vi "Loop.vi"(7 "Stop Button":bool, 8 "Inputs":T5 {"Color Pane" items=["Blue", "Red", "Green", "Saturation", "Value", "Intensity", "Luminance", "Hue", ""]}, 10 "Reference":T1, 11 "cam5":T6="cam5") -> (0 "Force Cluster":T3, 1 "Diameter Time":dbl, 2 "Force Time":dbl, 3 "Diameter Cluster":T4, 5 "Start Time":timestamp)   [LabVIEW 2020]
uses:
  StateControl.ctl
  <vilib>/vision/driver/NI_Vision_Acquisition_Software.lvlib
  <extravilib>/ChannelInstances/Tag-bool.lvlib
  <vilib>/DAQmx/create/channels.llb/DAQmx Create Channel (AI-Voltage-Basic).vi
  <vilib>/DAQmx/configure/timing.llb/DAQmx Timing (Sample Clock).vi
  <vilib>/DAQmx/write.llb/DAQmx Write (Counter Frequency 1Chan 1Samp).vi
  <vilib>/DAQmx/write.llb/DAQmx Write (Digital Bool 1Line 1Point).vi
  Inputs.ctl
  <vilib>/userDefined/High Color/IMAQdx.ctl
  ButtonReferences.ctl
  BR2.ctl
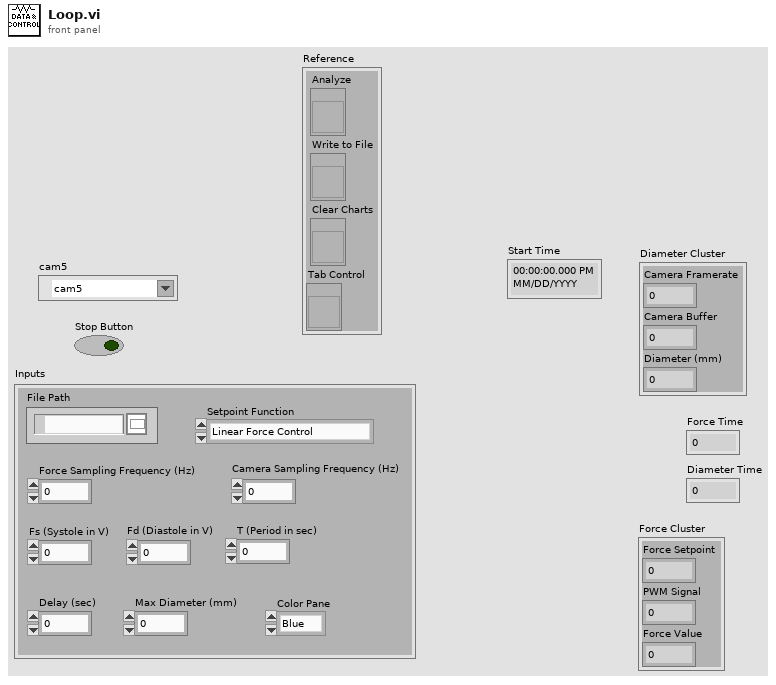
[diagram p1: front panel]
types:
  T1 = typedef "BR2.ctl" = cluster{"Analyze":refnum<vi>, "Write to File":T2, "Clear Charts":refnum<vi>, "Tab Control":refnum<vi>}
  T2 = typedef "ButtonReferences.ctl" = refnum<vi>
  T3 = cluster{"Force Setpoint":dbl, "PWM Signal":dbl, "Force Value":dbl}
  T4 = cluster{"Camera Framerate":dbl, "Camera Buffer":u32, "Diameter (mm)":dbl}
  T5 = typedef "Inputs.ctl" = cluster{"File Path":path, "Force Sampling Frequency (Hz)":dbl, "Camera Sampling Frequency (Hz)":dbl, "Fs (Systole in V)":dbl, "Fd (Diastole in V)":dbl, "T (Period in sec)":dbl, "Delay (sec)":dbl, "Setpoint Function":enum16{"Linear Force Control", "Sinusoidal Force Control", "Blood-Pressure Force Control"}, "Max Diameter (mm)":dbl, "Color Pane":i32}
  T6 = typedef "IMAQdx.ctl" = refnum<k21>
  T7 = typedef "StateControl.ctl" = enum16{"Initialze", "Wait for Event", "Acquire", "Shutdown"}
  T8 = enum8{"Enabled", "Disabled", "Disabled and Grayed Out"}
  T9 = typedef "Image Type" = u32
  T10 = typedef "IMAQ Image.ctl" = refnum<image>
  T11 = typedef "Tag-bool.lvlib/))Channel.ctl" = refnum<queue>
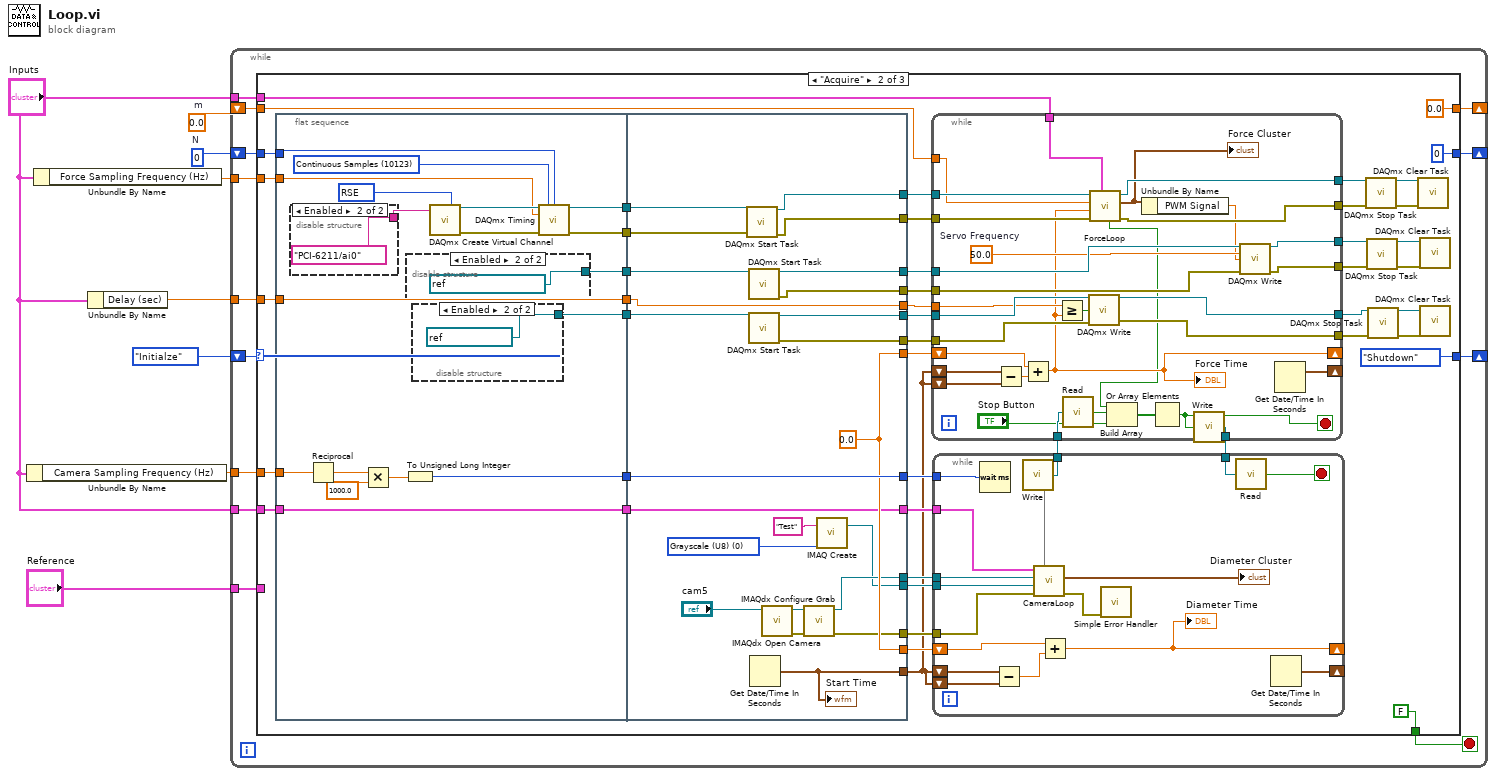
[diagram p0: block diagram]
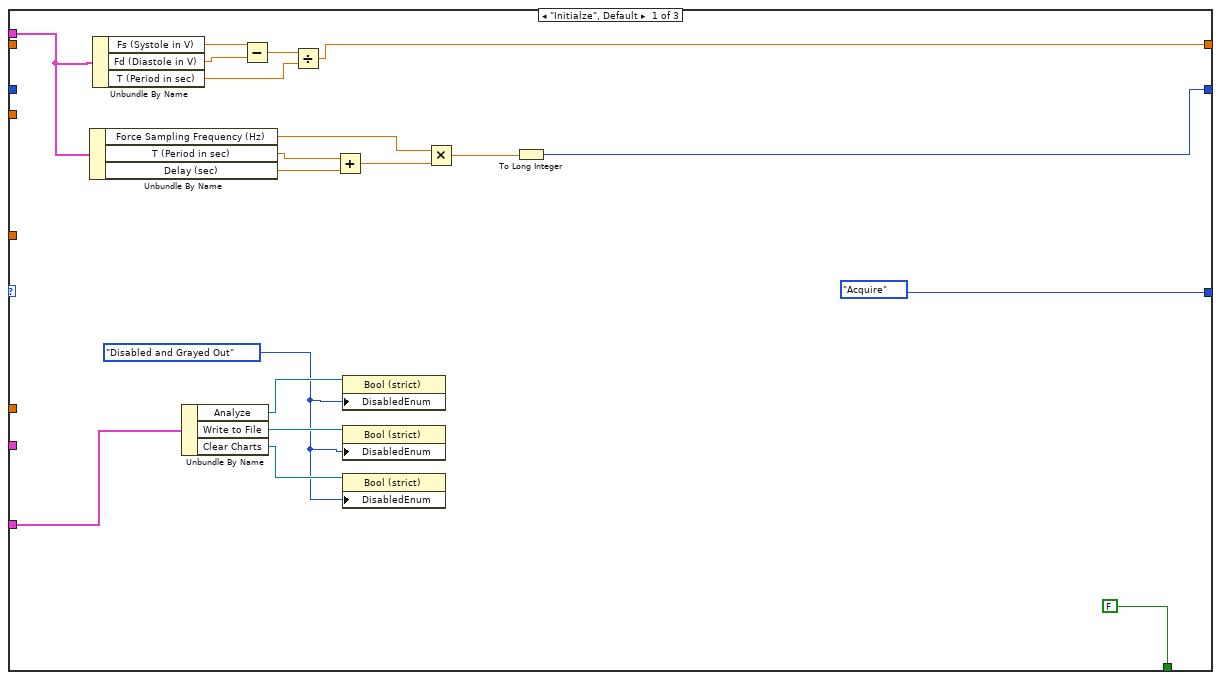
[diagram p2: hidden frame]
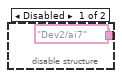
[diagram p3: hidden frame]
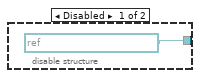
[diagram p4: hidden frame]
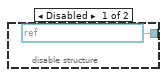
[diagram p5: hidden frame]
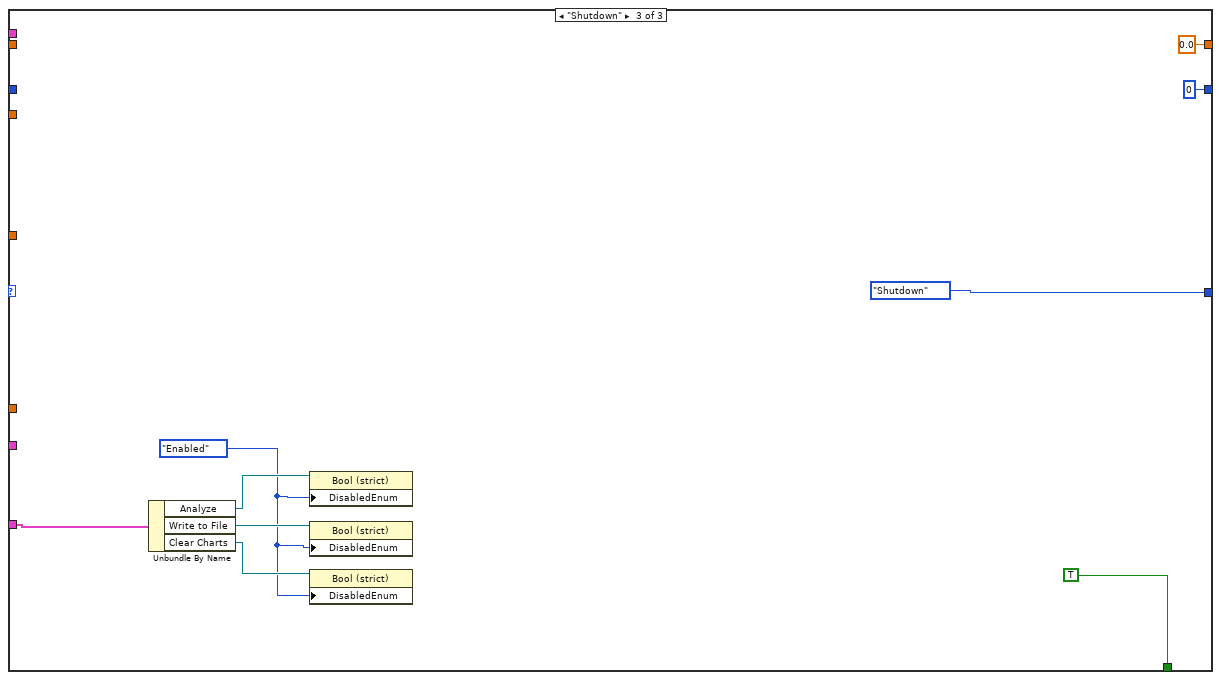
[diagram p6: hidden frame]
diagram:
  w4 = 0.0  # m
  w7 = 0  # N
  n1 = Unbundle By Name("Inputs") -> ("Camera Sampling Frequency (Hz)"=w5:dbl)
  n2 = Unbundle By Name("Inputs") -> ("Force Sampling Frequency (Hz)"=w6:dbl)
  n3 = Unbundle By Name("Inputs") -> ("Delay (sec)"=w2:dbl)
  n4 = while {
    shift-right: [w20] -> _
    shift-left: StateControl."Initialze" ("Enum") -> [w21]
    shift-right: [w16] -> _
    shift-left: w7 -> [w19]
    tunnel: w6 -> [w18]
    tunnel: "Inputs" -> [w17]
    tunnel: w5 -> [w15]
    shift-right: [w13] -> _
    shift-left: w4 -> [w14]
    tunnel: "Inputs" -> [w12]
    tunnel: w2 -> [w11]
    tunnel: "Reference" -> [w9]
    stop <- w10 stop-if-true
    n5 = case shown="\"Acquire\"" w21 {
      tunnel: [StateControl."Acquire" ("Enum") StateControl."Shutdown" ("Enum") StateControl."Shutdown" ("Enum")] -> w20
      tunnel: w19 -> [_ w82 _]
      tunnel: w18 -> [_ w81 _]
      tunnel: w17 -> [w33 w49 _]
      tunnel: [w34 0 0] -> w16
      tunnel: w15 -> [_ w79 _]
      tunnel: w14 -> [_ w76 _]
      tunnel: [w28 0.0 0.0] -> w13
      tunnel: w12 -> [_ w70 _]
      tunnel: w11 -> [_ w64 _]
      tunnel: [FALSE ("stop") FALSE ("stop") TRUE ("stop")] -> w10
      tunnel: w9 -> [w24 _ w184]
      frame "Initialze", Default {
        w22 = T8."Disabled and Grayed Out" ("Disabled")
        n6 = Unbundle By Name(w33) -> ("Force Sampling Frequency (Hz)"=w36:dbl, "T (Period in sec)"=w39:dbl, "Delay (sec)"=w38:dbl)
        n7 = Unbundle By Name(w33) -> ("Fs (Systole in V)"=w32:dbl, "Fd (Diastole in V)"=w31:dbl, "T (Period in sec)"=w29:dbl)
        n8 = Unbundle By Name(w24) -> ("Analyze"=w26:refnum<vi>, "Write to File"=w25:T2, "Clear Charts"=w23:refnum<vi>)
        n9 = Subtract(x=w32, y=w31) -> (x-y=w30:dbl)
        n10 = Divide(x=w30, y=w29) -> (x/y=w28:dbl)
        n11 = Add(x=w39, y=w38) -> (x+y=w37:dbl)
        n12 = property class="Bool (strict)"(reference=w26, "DisabledEnum"=w22) -> ()  [unwired: 1 in, 2 out]
        n13 = property class="Bool (strict)"(reference=w25, "DisabledEnum"=w22) -> ()  [unwired: 1 in, 2 out]
        n14 = property class="Bool (strict)"(reference=w23, "DisabledEnum"=w22) -> ()  [unwired: 1 in, 2 out]
        n15 = Multiply(x=w36, y=w37) -> (x*y=w35:dbl)
        n16 = To Long Integer(number=w35) -> (32bit integer=w34:i32)
      }
      frame "Acquire" {
        n17 = flat-sequence {
          tunnel: [w149] -> w86
          tunnel: [w148] -> w85
          tunnel: [w147] -> w84
          tunnel: [w146] -> w83
          tunnel: w82 -> [w145]
          tunnel: w81 -> [w144]
          tunnel: w79 -> [w143]
          tunnel: [w139] -> w78
          tunnel: w70 -> [w138]
          tunnel: [w138] -> w69
          tunnel: w64 -> [w137]
          tunnel: [w137] -> w63
          tunnel: w86 -> [w178]
          tunnel: w85 -> [w177]
          tunnel: w84 -> [w176]
          tunnel: w83 -> [w175]
          tunnel: w78 -> [w174]
          tunnel: [w174] -> w77
          tunnel: [w173] -> w42
          tunnel: [w172] -> w74
          tunnel: [w172] -> w73
          tunnel: [w171] -> w72
          tunnel: [w170] -> w71
          tunnel: w69 -> [w169]
          tunnel: [w169] -> w68
          tunnel: [w168] -> w67
          tunnel: w63 -> [w167]
          tunnel: [w167] -> w60
          tunnel: [w166] -> w62
          tunnel: [w165] -> w61
          tunnel: [w164] -> w59
          tunnel: [w163] -> w58
          tunnel: [w162] -> w48
          tunnel: [w161] -> w47
          frame #0 {
            w150 = 10083 items=["Default"=-1, "RSE"=10083, "NRSE"=10078, "Differential"=10106, "Pseudodifferential"=12529] ("input terminal configuration")
            w151 = 10123 items=["Finite Samples"=10178, "Continuous Samples"=10123, "Hardware Timed Single Point"=12522] ("sample mode")
            n18 = disable-structure shown="Enabled" {
              disable-tunnel: [tag "Dev2/ai7" ("physical channels") tag "PCI-6211/ai0" ("physical channels")] -> w154
              frame Disabled {
              }
              frame Enabled {
              }
            }
            n19 = Reciprocal(x=w143) -> (1/x=w142:dbl)
            n20 = Multiply(x=w142, y=1000.0) -> (x*y=w140:dbl)
            n21 = To Unsigned Long Integer(number=w140) -> (unsigned 32bit integer=w139:u32)
            n22 = disable-structure shown="Enabled" {
              disable-tunnel: [refnum<k21> "MyPulseOutputTask" ("DAQmx Task Name") refnum<k21> "MyPulseOutTask" ("DAQmx Task Name")] -> w147
              frame Disabled {
              }
              frame Enabled {
              }
            }
            n23 = disable-structure shown="Enabled" {
              disable-tunnel: [refnum<k21> "MyDigitalOutTask" ("DAQmx Task Name") refnum<k21> "SimDigOut" ("DAQmx Task Name")] -> w146
              frame Disabled {
              }
              frame Enabled {
              }
            }
            n24 = call-poly <vilib>:"DAQmx Create Virtual Channel.vi"("input terminal configuration"=w150, "physical channels"=w154) -> ("task out"=w152:refnum<k21>, "error out"=w153:errorcluster)  [unwired: 12 in]
            n25 = call-poly <vilib>:"DAQmx Timing.vi"("task/channels in"=w152, "sample mode"=w151, "samples per channel"=w145, "rate"=w144, "error in"=w153) -> ("task out"=w149:refnum<k21>, "error out"=w148:errorcluster)  [unwired: 9 in]
          }
          frame #1 {
            w172 = 0.0
            w179 = T9 0 items=["Grayscale (U8)", "Grayscale (I16)", "Grayscale (SGL)", "Complex (CSG)", "RGB (U32)", "HSL (U32)", "RGB (U64)", "Grayscale (U16)"] ("Image Type")
            n26 = call <vilib>:"DAQmx Start Task.vi"("task/channels in"=w178, "error in"=w177) -> ("task out"=w162:refnum<k21>, "error out"=w161:errorcluster)  [unwired: 12 in]
            n27 = call <vilib>:"DAQmx Start Task.vi"("task/channels in"=w176) -> ("task out"=w164:refnum<k21>, "error out"=w163:errorcluster)  [unwired: 13 in]
            n28 = call <vilib>:"DAQmx Start Task.vi"("task/channels in"=w175) -> ("task out"=w166:refnum<k21>, "error out"=w165:errorcluster)  [unwired: 13 in]
            n29 = Get Date/Time In Seconds() -> (seconds since 1Jan1904=w173:timestamp)
            "Start Time" <- w173
            n30 = call <vilib>:"IMAQdx Open Camera.vi"("Session In"="cam5") -> ("error out"=w183:errorcluster, "Session Out"=w182:T6)  [unwired: 9 in]
            n31 = call <vilib>:"IMAQdx Configure Grab.vi"("error in"=w183, "Session In"=w182) -> ("error out"=w168:errorcluster, "Session Out"=w171:T6)  [unwired: 8 in]
            n32 = call "IMAQ Create"("Image Name"="Test", "Image Type"=w179) -> ("New Image"=w170:T10)  [unwired: 3 in, 1 out]
          }
        }
        n33 = while {
          tunnel: w76 -> [w98]
          shift-right: [w115] -> _
          shift-left: w42 -> [w119]
          shift-left: w42 -> [w118]
          shift-right: [w97] -> _
          shift-left: w74 -> [w117]
          tunnel: w66 -> [w114]
          tunnel: [w113] -> w65
          tunnel: w62 -> [w112]
          tunnel: w61 -> [w111]
          tunnel: w60 -> [w109]
          tunnel: w59 -> [w108]
          tunnel: w58 -> [w107]
          tunnel: [w105] -> w53
          tunnel: [w104] -> w52
          tunnel: [w103] -> w51
          tunnel: [w102] -> w50
          tunnel: w49 -> [w101]
          tunnel: w48 -> [w100]
          tunnel: w47 -> [w99]
          tunnel: [w96] -> w44
          tunnel: [w95] -> w43
          stop <- w89 stop-if-true
          w106 = 50.0  # Servo Frequency
          n34 = Subtract(x=w119, y=w118) -> (x-y=w116:dbl)
          n35 = Add(x=w117, y=w116) -> (x+y=w97:dbl)
          "Force Time" <- w97
          n36 = Greater Or Equal?(x=w109, y=w97) -> (x >= y?=w110:bool)
          n37 = call <extravilib>:"Read.vi"("channel"=w114) -> ("element"=w92:bool)  [unwired: 1 in, 1 out]
          n38 = call-poly <vilib>:"DAQmx Write.vi"("task/channels in"=w112, "data"=w110, "error in"=w111) -> ("task out"=w105:refnum<k21>, "error out"=w104:errorcluster)  [unwired: 10 in, 1 out]
          n39 = call "ForceLoop.vi"("Inputs"=w101, "error in"=w99, "Time"=w97, "Slope"=w98, "task/channels in"=w100) -> ("error out"=w95:errorcluster, "Force Cluster"=w94:T3, "task out"=w96:refnum<k21>, "Time Exceeded?"=w91:bool)  [unwired: 3 in]
          "Force Cluster" <- w94
          n40 = Build Array(w91, w92, "Stop Button") -> (w90:bool[])
          n41 = Unbundle By Name(w94) -> ("PWM Signal"=w93:dbl)
          n42 = Or Array Elements(Boolean array=w90) -> (logical OR=w89:bool)
          n43 = call <extravilib>:"Write.vi"("element"=w89) -> ("channel"=w113:T11)  [unwired: 1 out]
          n44 = call-poly <vilib>:"DAQmx Write.vi"("task/channels in"=w108, "frequency"=w106, "duty cycle"=w93, "error in"=w107) -> ("task out"=w103:refnum<k21>, "error out"=w102:errorcluster)  [unwired: 9 in, 1 out]
          n45 = Get Date/Time In Seconds() -> (seconds since 1Jan1904=w115:timestamp)
        }
        n46 = while {
          tunnel: w77 -> [w136]
          shift-right: [w135] -> _
          shift-left: w42 -> [w133]
          shift-left: w42 -> [w134]
          shift-right: [w132] -> _
          shift-left: w73 -> [w131]
          tunnel: w72 -> [w129]
          tunnel: w71 -> [w128]
          tunnel: w68 -> [w127]
          tunnel: w67 -> [w126]
          tunnel: [w124] -> w66
          tunnel: w65 -> [w123]
          stop <- w122 stop-if-true
          n47 = Wait (ms)(milliseconds to wait=w136) -> ()  [unwired: 1 out]
          n48 = Subtract(x=w133, y=w134) -> (x-y=w130:dbl)
          n49 = call "CameraLoop.vi"("error in"=w126, "Image In"=w128, "Session In"=w129, "Inputs"=w127) -> ("error out"=w120:errorcluster, "Diameter Cluster"=→"Diameter Cluster":T4, 3:w125)  [unwired: 4 in]
          n50 = call <extravilib>:"Write.vi"("element"=w125) -> ("channel"=w124:T11)  [unwired: 1 out]
          n51 = Add(x=w131, y=w130) -> (x+y=w132:dbl)
          "Diameter Time" <- w132
          n52 = call <vilib>:"Simple Error Handler.vi"("error in (no error)"=w120) -> ()  [unwired: 4 in, 5 out]
          n53 = call <extravilib>:"Read.vi"("channel"=w123) -> ("element"=w122:bool)  [unwired: 1 in, 1 out]
          n54 = Get Date/Time In Seconds() -> (seconds since 1Jan1904=w135:timestamp)
        }
        n55 = call <vilib>:"DAQmx Stop Task.vi"("task/channels in"=w44, "error in"=w43) -> ("task out"=w46:refnum<k21>, "error out"=w45:errorcluster)  [unwired: 12 in]
        n56 = call <vilib>:"DAQmx Stop Task.vi"("task/channels in"=w51, "error in"=w50) -> ("task out"=w57:refnum<k21>, "error out"=w56:errorcluster)  [unwired: 12 in]
        n57 = call <vilib>:"DAQmx Stop Task.vi"("task/channels in"=w53, "error in"=w52) -> ("task out"=w55:refnum<k21>, "error out"=w54:errorcluster)  [unwired: 12 in]
        n58 = call <vilib>:"DAQmx Clear Task.vi"("task in"=w46, "error in"=w45) -> ()  [unwired: 13 in, 1 out]
        n59 = call <vilib>:"DAQmx Clear Task.vi"("task in"=w57, "error in"=w56) -> ()  [unwired: 13 in, 1 out]
        n60 = call <vilib>:"DAQmx Clear Task.vi"("task in"=w55, "error in"=w54) -> ()  [unwired: 13 in, 1 out]
      }
      frame "Shutdown" {
        w185 = T8."Enabled" ("Disabled")
        n61 = Unbundle By Name(w184) -> ("Analyze"=w188:refnum<vi>, "Write to File"=w187:T2, "Clear Charts"=w186:refnum<vi>)
        n62 = property class="Bool (strict)"(reference=w188, "DisabledEnum"=w185) -> ()  [unwired: 1 in, 2 out]
        n63 = property class="Bool (strict)"(reference=w187, "DisabledEnum"=w185) -> ()  [unwired: 1 in, 2 out]
        n64 = property class="Bool (strict)"(reference=w186, "DisabledEnum"=w185) -> ()  [unwired: 1 in, 2 out]
      }
    }
  }
